vi "path steer7.vi"(11 "lane":bool) -> (2 "curve vel limit":dbl=3.2139390725243686, 3 "handle":dbl=-81.96459499192818)   [LabVIEW 2015]
uses:
  G_ALL.vi
  G_LCM.vi
  <vilib>/Analysis/polynomials.llb/Scalar Polynomial Evaluation (DBL).vi
  <vilib>/Analysis/polynomials.llb/nth Derivative of Polynomial (DBL).vi
  <vilib>/Analysis/polynomials.llb/1D Polynomial Evaluation (DBL).vi
  <vilib>/Analysis/NI_AALPro.lvlib
  G_SEN.vi
  <vilib>/gmath/NI_Gmath.lvlib
panel:
  out "Waveform Chart 2":dynamicdata(graph)
  in  "lpf gain 2":dbl=0.88 format="%#_13g"
  in  "parking stop":bool=TRUE
  out "cy":dbl
  out "cx":dbl
  out "slope ab":dbl
  out "slope bc":dbl
  out "current":i32
  in  "speed gain":dbl=0.3 format="%#_13g"
  in  "lpf gain":dbl=0.1 format="%#_13g"
  out "Waveform Chart":dbl(graph)=3.2139390725243686
  in  "index (row)":i32
  out "dist speed":dbl[](array[numeric])=[-2.893089960514653, -2.3904015790595508, -1.881068928132613, -1.37618634654772, -0.8742713561658589, -0.3723658755970851, 0.1388818221238658, 0.6401970171432404, 1.1461801054227339, 1.6534687725008643, 2.1616153665314632, 2.66800643713298, 3.175087235872203, 3.683904013545636, 4.1920491404702815, 4.703688631377526, 5.208864123676872, 5.719321128099619, 6.224971964952173, 6.729181230795628, 7.2363172303323795, 7.739934572021128, 8.247038660118557, 8.752204204665103, 9.255845634255843, 9.765210087355028, 10.274718584659908, 10.78117636416095, 11.281375299651366, 11.781461553901512, 12.293088227883759, 12.79457373850707, 13.302719176130964, 13.812473318001016, 14.318113179991025, 14.83081141605283, 15.340843713390877, 15.852065999952396, 16.364391250745, 16.8738363825444, 17.383376701480152, 17.890443538120152, 18.401927893044, 18.911251065570802, 19.420871980672878, 19.927741491376995, 20.442181893066248, 20.954251161353227, 21.455793255420453, 21.973813140636935, 22.47769405993468, 22.987685957840586, 23.50066957065988, 24.01168868408926, 24.517992353494144]
  out "Polynomial Coefficients 2":dbl[](array[numeric])
  out "R0":dbl=26.83387719970357
  out "handle 2":dbl=81.96459499192818
  out "dist":dbl[](array[numeric])=[-3.4007239355103813, -2.893089960514653, -2.3904015790595508, -1.881068928132613, -1.37618634654772, -0.8742713561658589, -0.3723658755970851, 0.1388818221238658, 0.6401970171432404, 1.1461801054227339, 1.6534687725008643, 2.1616153665314632, 2.66800643713298, 3.175087235872203, 3.683904013545636, 4.1920491404702815, 4.703688631377526, 5.208864123676872, 5.719321128099619, 6.224971964952173]
  in  "ap[g]":dbl=0.01 format="%#_13g"
  in  "mu":dbl=0.35 format="%#_13g"
  in  "an[g]":dbl=-0.03 format="%#_13g"
  out "Waveform Graph 2":dynamicdata(graph)=[{"t0"=timestamp(3559051319.3986335 s since 1904-01-01), "dt"=1.0, "Y"=[12.201099406852837, 18.19581647475159, 7.659888709456787, 6.442363646204152, 5.714419173702362, 7.179343934552439, 4.440534485019003, 4.39078441294489, 3.356713814067408, 2.401942511989647, 2.947435527157797, 2.405147000486268, 2.4253719977268635, 2.206819680096971, 2.0623492643882435, 1.9270030620983392, 1.8994447737647506, 1.8, 1.8, 1.8, 1.8, 1.8, 1.8, 2.1782596057309664, 2.252935408002384, 2.211867158231172, 2.2822368344295345, 2.820696071361234, 3.770354448612146, 2.5415686609617323, 9.592181945625502, 6.158409445479877, 5.390039216536413, 5.524972901149052, 13.273555614419179, 5.975286485301752, 11.57649163445339, 9.01145671123187, 9.660936533884865, 7.724510571264461, 5.533992586139264, 6.25966127157872, 14.880677288421989, 7.369567618162387, 13.568928447863307, 21.814825265892647, 18.32662456942843, 11.069099853071005, 65.39630065395748, 8.723651409692232, 11.138954896953177, 34.68633250782535, 14.254469597416035, 11.910088090354131, 13.122894121811795]}, {"t0"=timestamp(3559051319.3986335 s since 1904-01-01), "dt"=1.0, "Y"=[4.162943567044335, 4.006480657019834, 3.8414555364164134, 3.6705571026990116, 3.4923837272772165, 3.304621450941619, 3.101700634836984, 2.8889144351091893, 2.6569224873325505, 2.401942511989647, 2.659390719977461, 2.405147000486268, 2.4253719977268635, 2.206819680096971, 2.0623492643882435, 1.9270030620983392, 1.8994447737647506, 1.8, 1.8, 1.8, 1.8, 1.8, 1.8, 2.1782596057309664, 2.252935408002384, 2.211867158231172, 2.2822368344295345, 2.820696071361234, 2.780497542086646, 2.5415686609617323, 5.623145371472975, 5.508594247501762, 5.390039216536413, 5.524972901149052, 6.083396505782966, 5.975286485301752, 5.984875001532974, 5.8752716781758645, 5.763341152167903, 5.649841467554542, 5.533992586139264, 6.25966127157872, 7.456916882616871, 7.369567618162387, 9.088101570636532, 9.016914477587346, 8.944084767926125, 8.8709969665068, 8.798823217737656, 8.723651409692232, 11.138954896953177, 12.018901085380875, 11.964513913766247, 11.910088090354131, 13.122894121811795]}, {"t0"=timestamp(0 s since 1904-01-01), "dt"=1.0, "Y"=[4.162943567044335, 4.006480657019834, 3.8414555364164134, 3.6705571026990116, 3.4923837272772165, 3.304621450941619, 3.101700634836984, 2.8889144351091893, 2.6569224873325505, 2.401942511989647, 2.659390719977461, 2.405147000486268, 2.4253719977268635, 2.206819680096971, 2.0623492643882435, 1.9270030620983392, 1.8994447737647506, 1.8, 1.8, 1.8, 1.8, 1.8, 1.8, 2.1782596057309664, 2.252935408002384, 2.211867158231172, 2.2822368344295345, 2.820696071361234, 2.780497542086646, 2.5415686609617323, 5.623145371472975, 5.508594247501762, 5.390039216536413, 5.524972901149052, 6.083396505782966, 5.975286485301752, 5.984875001532974, 5.8752716781758645, 5.763341152167903, 5.649841467554542, 5.533992586139264, 6.25966127157872, 7.456916882616871, 7.369567618162387, 9.088101570636532, 9.016914477587346, 8.944084767926125, 8.8709969665068, 8.798823217737656, 8.723651409692232, 11.138954896953177, 12.018901085380875, 11.964513913766247, 11.910088090354131, 13.122894121811795]}]
  out "map_track for speed":dbl[][](array[numeric])=[[0.11349876041351359, -3.3998372416388567], [0.10142427488084116, -2.8923468876723155], [0.08838339602237211, -2.3898276897021793], [0.07566482613937353, -1.8806538615448463], [0.06028455243766717, -1.376005599516048], [0.0488631758884196, -0.8742205760969111], [0.04234520267579428, -0.3723574199973909], [0.038899869961946, 0.1388786684269922], [0.04370378366690808, 0.6401708458748642], [0.056953881218304414, 1.1459804153174877], [0.08472623749133856, 1.6525082901407298], [0.14087522942915354, 2.1575431916369188], [0.21546998499325254, 2.6584099791436198], [0.3179687305625989, 3.155023454199139], [0.44800644132001843, 3.6469428653052116], [0.6101750776411523, 4.128516123918072], [0.8099098158192999, 4.599558588055575], [1.0468148112307838, 5.045740502938923], [1.3255371094151536, 5.4733854887145865], [1.6426512363159849, 5.867240029541034], [1.9985777122494781, 6.224372116438809], [2.393384520275489, 6.5426715138030715], [2.816110574573037, 6.816410641199336], [3.267091466034361, 7.048295939788691], [3.738316452139705, 7.23033780274067], [4.219304825636487, 7.3796859669782116], [4.714356791323436, 7.499584663178458], [5.216398310074203, 7.586493939301898], [5.719828055076203, 7.641792892857529], [6.218830226700244, 7.6763733465884485], [6.718368390858731, 7.699780273749206], [7.229992817877207, 7.698263959746944], [7.731478256454141, 7.698532772738272], [8.239607735597689, 7.694505589692504], [8.749269272570775, 7.684789475041773], [9.254687125600576, 7.669807356632795], [9.767131481073555, 7.653674662971492], [10.277036204891097, 7.642267780992534], [10.788156814263154, 7.632072245090674], [11.300416991351074, 7.623906856578211], [11.809822584072345, 7.617559855837815], [12.319350308624628, 7.613977324090475], [12.826414003897163, 7.615762192897625], [13.337862856989585, 7.621788468887832], [13.847141338275545, 7.628535510597585], [14.35666821837679, 7.638325074620945], [14.8634605074283, 7.647172483245015], [15.377816289134199, 7.6565029020949416], [15.889810107971169, 7.665292953101379], [16.391253932531534, 7.675220839664499], [16.909171541171744, 7.685514145261032], [17.412991119838455, 7.6933762686663645], [17.92293988059403, 7.700009317250687], [18.43587828140128, 7.706819897140418], [18.946840832903064, 7.714422873724447], [19.45310431820556, 7.720801674725955], [19.97546574871732, 7.728375286190201]]
  out "Polynomial Coefficients":dbl[](array[numeric])=[0.03615792236483369, -0.0013391473415595393, 0.015775244563062195, 0.003058081181776752, 0.00017869743224815146, 3.406886139257993e-05]
  out "XY Graph":cluster{"Y":dbl[], "Y":dbl[]}[](graph)=[{"Y"=[0.11349876041351359, 0.10142427488084116, 0.08838339602237211, 0.07566482613937353, 0.06028455243766717, 0.0488631758884196, 0.04234520267579428, 0.038899869961946, 0.04370378366690808, 0.056953881218304414, 0.08472623749133856, 0.14087522942915354, 0.21546998499325254, 0.3179687305625989, 0.44800644132001843, 0.6101750776411523, 0.8099098158192999, 1.0468148112307838, 1.3255371094151536, 1.6426512363159849, 1.9985777122494781, 2.393384520275489, 2.816110574573037, 3.267091466034361, 3.738316452139705, 4.219304825636487, 4.714356791323436, 5.216398310074203, 5.719828055076203, 6.218830226700244, 6.718368390858731, 7.229992817877207, 7.731478256454141, 8.239607735597689, 8.749269272570775, 9.254687125600576, 9.767131481073555, 10.277036204891097, 10.788156814263154, 11.300416991351074, 11.809822584072345, 12.319350308624628, 12.826414003897163, 13.337862856989585, 13.847141338275545, 14.35666821837679, 14.8634605074283, 15.377816289134199, 15.889810107971169, 16.391253932531534, 16.909171541171744, 17.412991119838455, 17.92293988059403, 18.43587828140128, 18.946840832903064, 19.45310431820556, 19.97546574871732], "Y"=[-3.3998372416388567, -2.8923468876723155, -2.3898276897021793, -1.8806538615448463, -1.376005599516048, -0.8742205760969111, -0.3723574199973909, 0.1388786684269922, 0.6401708458748642, 1.1459804153174877, 1.6525082901407298, 2.1575431916369188, 2.6584099791436198, 3.155023454199139, 3.6469428653052116, 4.128516123918072, 4.599558588055575, 5.045740502938923, 5.4733854887145865, 5.867240029541034, 6.224372116438809, 6.5426715138030715, 6.816410641199336, 7.048295939788691, 7.23033780274067, 7.3796859669782116, 7.499584663178458, 7.586493939301898, 7.641792892857529, 7.6763733465884485, 7.699780273749206, 7.698263959746944, 7.698532772738272, 7.694505589692504, 7.684789475041773, 7.669807356632795, 7.653674662971492, 7.642267780992534, 7.632072245090674, 7.623906856578211, 7.617559855837815, 7.613977324090475, 7.615762192897625, 7.621788468887832, 7.628535510597585, 7.638325074620945, 7.647172483245015, 7.6565029020949416, 7.665292953101379, 7.675220839664499, 7.685514145261032, 7.6933762686663645, 7.700009317250687, 7.706819897140418, 7.714422873724447, 7.720801674725955, 7.728375286190201]}, {"Y"=[0.11127739316480087, 0.10361692506575307, 0.0908884914373908, 0.07556394971539812, 0.06037459789185977, 0.04742882065356524, 0.03868911291226688, 0.03628446458426678, 0.04260160497064784, 0.06031835031844553, 0.09257618876938067, 0.14288063799816245, 0.21498550882016326, 0.3133602690293894, 0.44300969189444267, 0.607484992736191, 0.8114301214735165, 1.0511320562375182, 1.3305918725474135, 1.6376613473029409, 1.9629799067769196, 2.2950444233922735, 2.6156651813619924, 2.9148313405818387, 3.1686664277537977, 3.3900852782615782, 3.576818603835668, 3.7173442133091044, 3.809077950572423, 3.867374654316165, 3.907246206986835, 3.9046531883929876, 3.905112777752115, 3.898232126569368, 3.8816723523358934, 3.856249915036759, 3.829027163652526, 3.809873646729178, 3.79282033229891, 3.779207635636962, 3.768653959202114, 3.762707611314233, 3.7656692101174953, 3.775682543110717, 3.786919264560898, 3.8032715749983694, 3.8180996271049827, 3.8337882452990133, 3.848616328842317, 3.865420072795456, 3.88290546839812, 3.8963043998905627, 3.9076380118640244, 3.9193029379730002, 3.932358601774901, 3.943339494877334, 3.9564096926462176], "Y"=[-3.3998372416388567, -2.8923468876723155, -2.3898276897021793, -1.8806538615448463, -1.376005599516048, -0.8742205760969111, -0.3723574199973909, 0.1388786684269922, 0.6401708458748642, 1.1459804153174877, 1.6525082901407298, 2.1575431916369188, 2.6584099791436198, 3.155023454199139, 3.6469428653052116, 4.128516123918072, 4.599558588055575, 5.045740502938923, 5.4733854887145865, 5.867240029541034, 6.224372116438809, 6.5426715138030715, 6.816410641199336, 7.048295939788691, 7.23033780274067, 7.3796859669782116, 7.499584663178458, 7.586493939301898, 7.641792892857529, 7.6763733465884485, 7.699780273749206, 7.698263959746944, 7.698532772738272, 7.694505589692504, 7.684789475041773, 7.669807356632795, 7.653674662971492, 7.642267780992534, 7.632072245090674, 7.623906856578211, 7.617559855837815, 7.613977324090475, 7.615762192897625, 7.621788468887832, 7.628535510597585, 7.638325074620945, 7.647172483245015, 7.6565029020949416, 7.665292953101379, 7.675220839664499, 7.685514145261032, 7.6933762686663645, 7.700009317250687, 7.706819897140418, 7.714422873724447, 7.720801674725955, 7.728375286190201]}]
  out "ref":dbl[](array[numeric])=[91.349795796563, 0.0013391465410557935, 0.021526577035807966]
  in  "gain":dbl[](array[numeric])=[0.7, -1400.0, 750.0]
  out "path end":bool
  out "map_track for steering":dbl[][](array[numeric])=[[0.11349876041351359, -3.3998372416388567], [0.10142427488084116, -2.8923468876723155], [0.08838339602237211, -2.3898276897021793], [0.07566482613937353, -1.8806538615448463], [0.06028455243766717, -1.376005599516048], [0.0488631758884196, -0.8742205760969111], [0.04234520267579428, -0.3723574199973909], [0.038899869961946, 0.1388786684269922], [0.04370378366690808, 0.6401708458748642], [0.056953881218304414, 1.1459804153174877], [0.08472623749133856, 1.6525082901407298], [0.14087522942915354, 2.1575431916369188], [0.21546998499325254, 2.6584099791436198], [0.3179687305625989, 3.155023454199139], [0.44800644132001843, 3.6469428653052116], [0.6101750776411523, 4.128516123918072], [0.8099098158192999, 4.599558588055575], [1.0468148112307838, 5.045740502938923], [1.3255371094151536, 5.4733854887145865], [1.6426512363159849, 5.867240029541034]]
  in  "control point":dbl=0.3 format="%#_13g"
  out "R_new":dbl=26.837045395498738
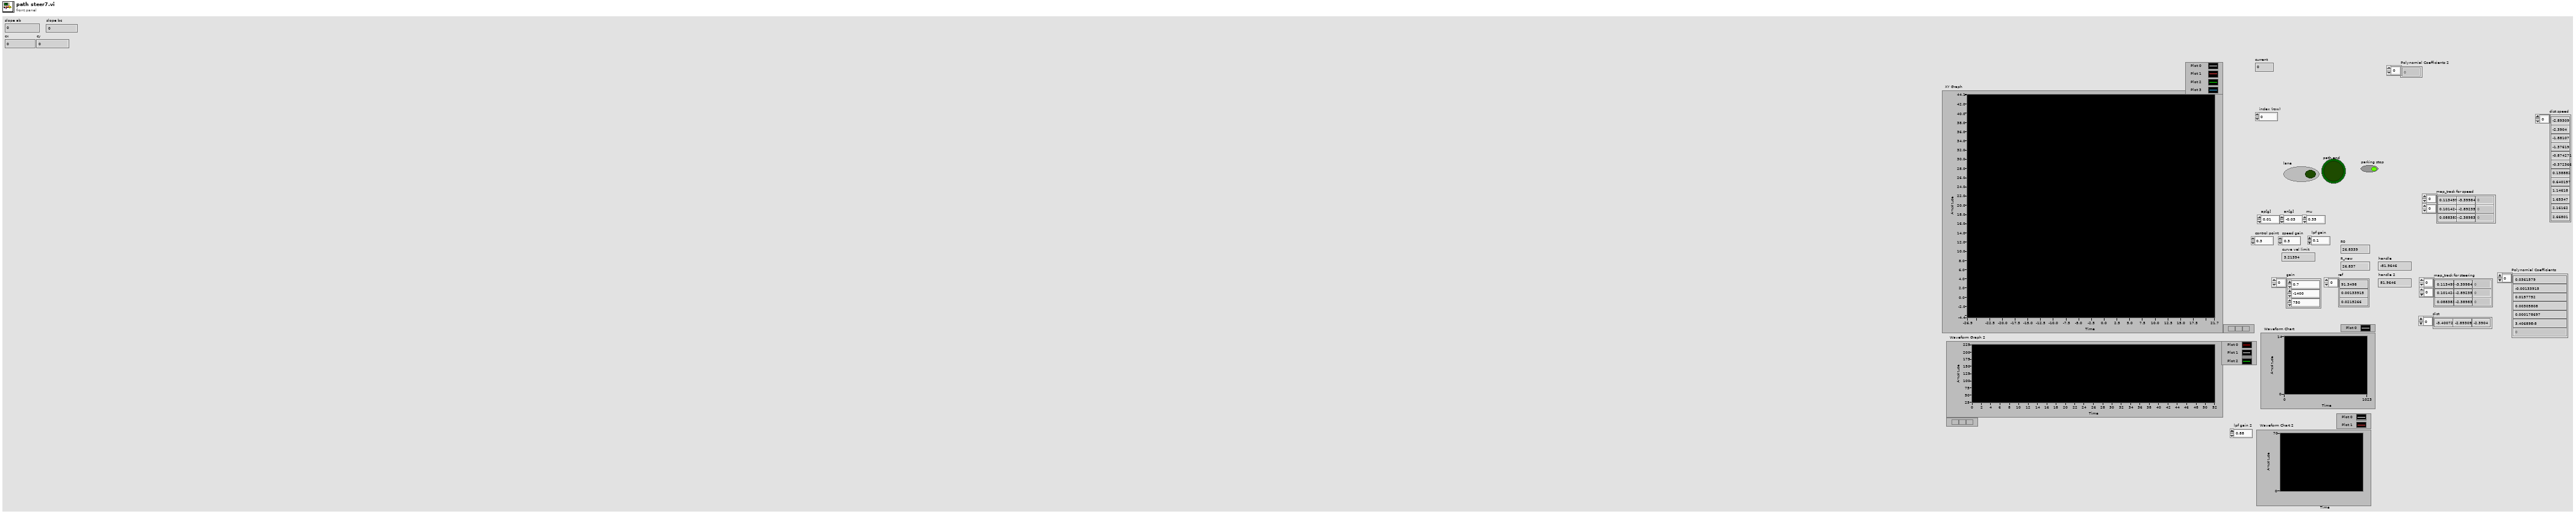
[diagram p1: front panel]
types:
  T1 = cluster{"Steer_input":dbl, "Steer_output":dbl, "VS_des":dbl, "VS_can":dbl, "heading":dbl, "auto":bool, "run":bool, "x":dbl, "y":dbl, "slam_y":dbl, "slam_x":dbl, "slam_heading":dbl}
  T2 = cluster{"C_Wheel base":dbl, "ratio_steer":dbl, "Overall width":dbl, "af":dbl, "turn radius":dbl, "eval":dbl, "ap":dbl, "an":dbl, "Vmax":dbl, "mu":dbl, "Vlast":dbl}
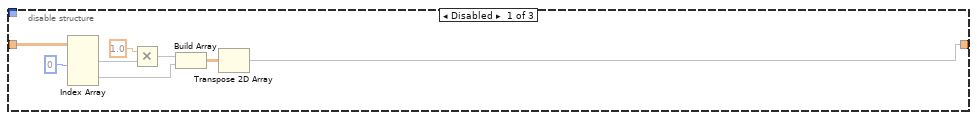
[diagram p2: hidden frame]
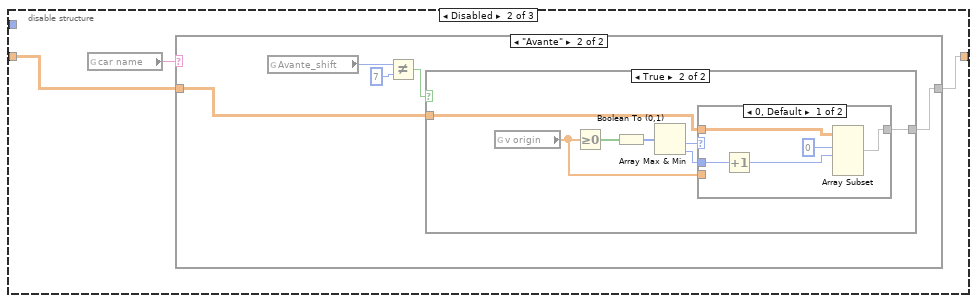
[diagram p3: hidden frame]
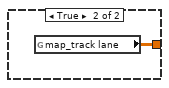
[diagram p7: hidden frame]
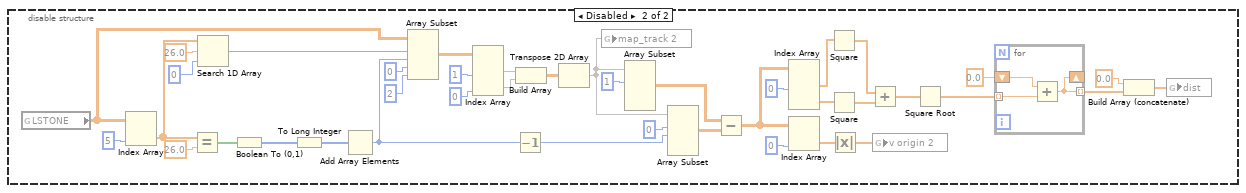
[diagram p8: hidden frame]
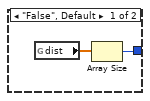
[diagram p11: hidden frame]
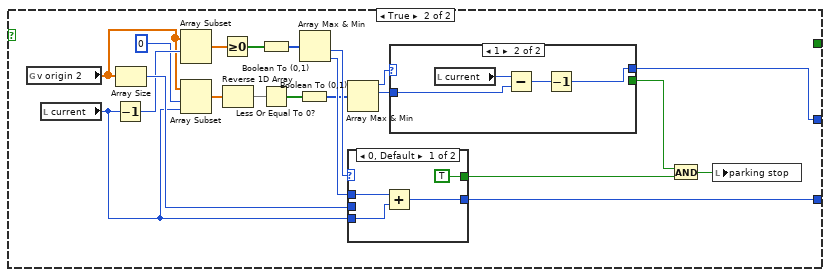
[diagram p13: hidden frame]
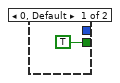
[diagram p14: hidden frame]
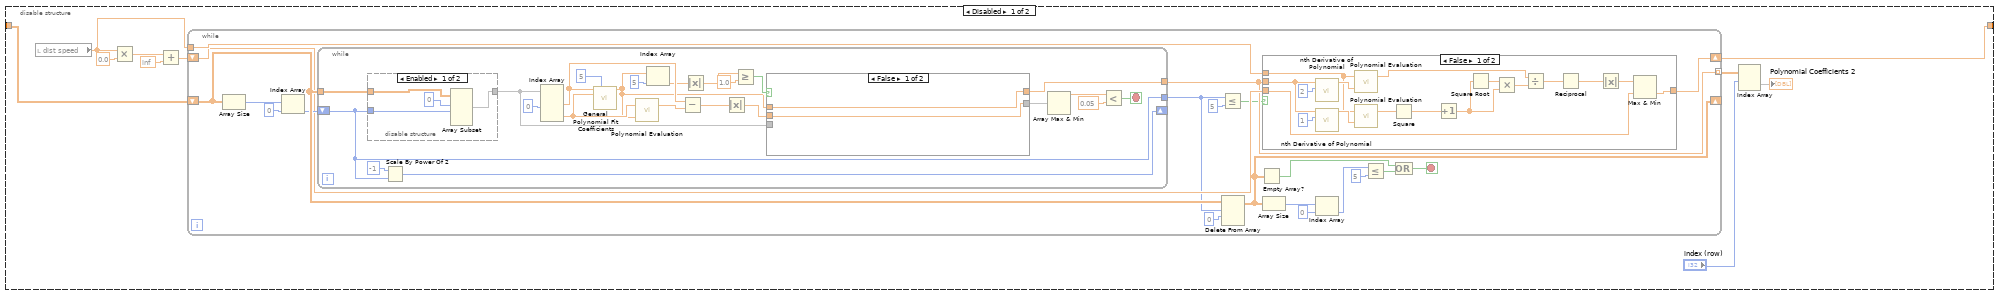
[diagram p16: hidden frame]
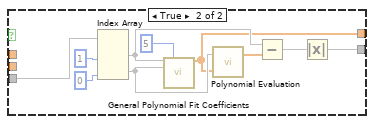
[diagram p18: hidden frame]
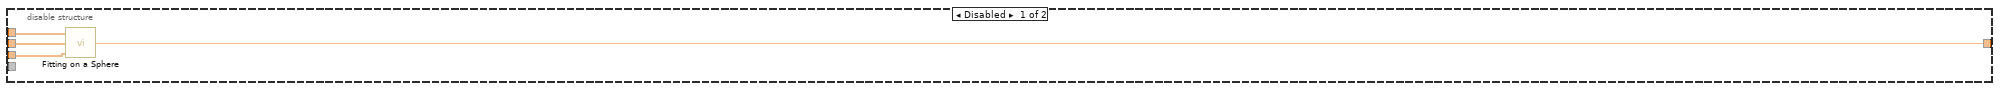
[diagram p20: hidden frame]
diagram:
  n1 = flat-sequence {
    tunnel: [w265] -> w2
    tunnel: w2 -> [w518]
    tunnel: [w633] -> w6
    tunnel: w6 -> [w644]
    tunnel: [w644] -> w5
    tunnel: [w638] -> w4
    tunnel: [w634] -> w3
    tunnel: [w635] -> w1
    tunnel: w5 -> [w696]
    tunnel: w4 -> [w694]
    tunnel: w3 -> [w675]
    tunnel: w1 -> [w671]
    frame #0 {
      n2 = disable-structure shown="Enabled" {
        frame Enabled {
          n3 = case shown="False" "lane" {
            tunnel: [w95 w138] -> w33
            tunnel: [w97 _] -> w66
            frame False {
              n4 = global read "G_ALL.vi" "current idx"() -> (w98:i32)
              n5 = Subtract(x=w98, y=2) -> (x-y=w105:i32)
              n6 = global read "G_ALL.vi" "map_track"() -> (w96:dbl[][])
              n7 = Max & Min(x=w105, y=0) -> (max(x,y)=w93:i32)  [unwired: 1 out]
              n8 = disable-structure shown="Enabled" {
                disable-tunnel: w96 -> [w114 w116 w137]
                disable-tunnel: [w107 w115 w137] -> w95
                disable-tunnel: w93 -> [_ _ _]
                frame Disabled {
                  n9 = Index Array(array=w114, index (col) #1=0 ("disabled index (col)")) -> (element #1=w112:dbl[], element #2=w109:dbl[])  [unwired: 3 in]
                  n10 = Multiply(x=1.0, y=w112) -> (x*y=w110:dbl[])
                  n11 = Build Array(w110, w109) -> (w108:dbl[][])
                  n12 = Transpose 2D Array(2D array=w108) -> (transposed array=w107:dbl[][])
                }
                frame Disabled {
                  n13 = global read "G_LCM.vi" "car name"() -> (w117:string)
                  n14 = case shown="\"Avante\"" w117 {
                    tunnel: [w118 w120] -> w115
                    tunnel: w116 -> [w118 w119]
                    frame Default {
                    }
                    frame "Avante" {
                      n15 = global read "G_ALL.vi" "Avante_shift"() -> (w122:u8)
                      n16 = Not Equal?(x=w122, y=u8 7) -> (x != y?=w121:bool)
                      n17 = case shown="True" w121 {
                        tunnel: [_ w126] -> w120
                        tunnel: w119 -> [_ w125]
                        frame False {
                        }
                        frame True {
                          n18 = global read "G_ALL.vi" "v origin"() -> (w127:dbl[])
                          n19 = Greater Or Equal To 0?(x=w127) -> (x >= 0?=w130:bool[])
                          n20 = Boolean To (0,1)(Boolean=w130) -> (0, 1=w129:i16[])
                          n21 = Array Max & Min(array=w129) -> (min value=w128:i16, min index (indices)=w124:i32)  [unwired: 2 out]
                          n22 = case shown="0, Default" w128 {
                            tunnel: w127 -> [_ _]
                            tunnel: [w132 w136] -> w126
                            tunnel: w125 -> [w134 w136]
                            tunnel: w124 -> [w135 _]
                            frame 0, Default {
                              n23 = Increment(x=w135) -> (x+1=w133:i32)
                              n24 = Array Subset(array=w134, index (row)=0 ("index"), length (row)=w133) -> (w132:dbl[][])  [unwired: 2 in]
                            }
                            frame 1 {
                            }
                          }
                        }
                      }
                    }
                  }
                }
                frame Enabled {
                }
              }
              n25 = Array Subset(array=w95, index (row)=w93, length (row)=5 ("length")) -> (w102:dbl[][])  [unwired: 2 in]
              n26 = Index Array(array=w102, index (col)=1 ("disabled index (col)")) -> (element=w100:dbl[])  [unwired: 1 in]
              n27 = Threshold 1D Array(2:0.0 ("threshold y"), 3:w100) -> (0:w94:dbl)  [unwired: 1 in]
              n28 = Add(x=w93, y=w94) -> (x+y=w97:dbl)
            }
            frame True {
              n29 = global read "G_ALL.vi" "map_track lane"() -> (w138:dbl[][])
            }
          }
          n30 = Round Toward -Infinity(1:w66) -> (0:w62:dbl)
          n31 = Index Array(array=w33, index (col) #1=0 ("disabled index (col)")) -> (element #1=w25:dbl[], element #2=w26:dbl[])  [unwired: 3 in]
          n32 = Equal?(x=w62, y=w66) -> (x = y?=w63:bool)
          n33 = To Long Integer(number=w62) -> (32bit integer=w64:i32)
          n34 = Interpolate 1D Array(1:w66, 2:w25) -> (0:w27:dbl)
          n35 = Interpolate 1D Array(1:w66, 2:w26) -> (0:w28:dbl)
          n36 = Increment(x=w64) -> (x+1=w65:i32)
          n37 = Round Toward +Infinity(x=w66) -> (ceil(x): smallest int >= x=w61:dbl)
          n38 = Select(t=w64, s=w63, f=w65) -> (s? t:f=w21:i32)
          n39 = global read "G_ALL.vi" "CARDATA"() -> (w31:T1)
          n40 = Array Subset(array=w33, index (row)=0 ("index"), length (row)=w21) -> (w35:dbl[][])  [unwired: 2 in]
          n41 = Unbundle By Name(w31) -> ("VS_can"=w67:dbl)
          n42 = Index Array(array=w35, index (col) #1=0 ("disabled index (col)")) -> (element #1=w37:dbl[], element #2=w38:dbl[])  [unwired: 3 in]
          n43 = Reverse 1D Array(array=w37) -> (reversed array=w39:dbl[])
          n44 = Reverse 1D Array(array=w38) -> (reversed array=w40:dbl[])
          n45 = Multiply(x=2.0, y=w67) -> (x*y=w68:dbl)
          n46 = Build Array(w39, w40) -> (w59:dbl[][])
          n47 = To Long Integer(number=w61) -> (32bit integer=w13:i32)
          n48 = Max & Min(x=w68, y=25.0) -> (max(x,y)=w32:dbl)  [unwired: 1 out]
          n49 = Array Subset(array=w33, index (row)=w13) -> (w57:dbl[][])  [unwired: 3 in]
          n50 = Transpose 2D Array(2D array=w59) -> (transposed array=w60:dbl[][])
          n51 = Build Array(w27, w28) -> (w42:dbl[])
          n52 = for {
            tunnel: w60 -> [w75] mode=indexing
            shift-right: [w75] -> _
            shift-left: w42 -> [w82]
            shift-right: [w74] -> _
            shift-left: 0.0 -> [w77]
            tunnel: 15.0 ("y") -> [w76]
            tunnel: [w74] -> w46 mode=indexing
            stop <- w73 stop-if-true
            n53 = Subtract(x=w75, y=w82) -> (x-y=w81:dbl[])
            n54 = Square(x=w81) -> (x^2=w80:dbl[])
            n55 = Add Array Elements(numeric array=w80) -> (sum=w79:dbl)
            n56 = Square Root(x=w79) -> (sqrt(x)=w78:dbl)
            n57 = Add(x=w77, y=w78) -> (x+y=w74:dbl)
            n58 = Greater Or Equal?(x=w74, y=w76) -> (x >= y?=w73:bool)
          }
          n59 = for {
            tunnel: w57 -> [w85] mode=indexing
            shift-right: [w85] -> _
            shift-left: w42 -> [w92]
            shift-right: [w84] -> _
            shift-left: 0.0 -> [w87]
            tunnel: w32 -> [w86]
            tunnel: [w84] -> w58 mode=indexing
            tunnel: [w83] -> w71
            stop <- w83 stop-if-true
            n60 = Subtract(x=w85, y=w92) -> (x-y=w91:dbl[])
            n61 = Square(x=w91) -> (x^2=w90:dbl[])
            n62 = Add Array Elements(numeric array=w90) -> (sum=w89:dbl)
            n63 = Square Root(x=w89) -> (sqrt(x)=w88:dbl)
            n64 = Add(x=w87, y=w88) -> (x+y=w84:dbl)
            n65 = Greater Or Equal?(x=w84, y=w86) -> (x >= y?=w83:bool)
          }
          n66 = global read "G_ALL.vi" "v origin"() -> (w14:dbl[])
          n67 = Array Subset(array=w14, index=0, length=w21) -> (w19:dbl[])
          n68 = Negate(x=w46) -> (-x=w44:dbl[])
          n69 = Not(x=w71) -> (.not. x?=→"path end":bool)
          n70 = Array Size(array=w46) -> (size(s)=w16:i32)
          n71 = Array Size(array=w58) -> (size(s)=w12:i32)
          n72 = Reverse 1D Array(array=w19) -> (reversed array=w18:dbl[])
          n73 = Array Subset(array=w14, index=w13, length=w12) -> (w11:dbl[])
          n74 = Reverse 1D Array(array=w44) -> (reversed array=w45:dbl[])
          n75 = Array Subset(array=w60, index (row)=0 ("index"), length (row)=w16) -> (w52:dbl[][])  [unwired: 2 in]
          n76 = Array Subset(array=w57, index (row)=0 ("index"), length (row)=w12) -> (w70:dbl[][])  [unwired: 2 in]
          n77 = Build Array (concatenate)(w45, w58) -> (w22:dbl[])
          n78 = Array Subset(array=w18, index=0, length=w16) -> (w15:dbl[])
          n79 = global write "G_ALL.vi" "dist"(w22) -> ()
          n80 = Reverse 1D Array(array=w15) -> (reversed array=w8:dbl[])
          n81 = Index Array(array=w52, index (col) #1=0 ("disabled index (col)")) -> (element #1=w53:dbl[], element #2=w54:dbl[])  [unwired: 3 in]
          n82 = Reverse 1D Array(array=w53) -> (reversed array=w50:dbl[])
          n83 = Reverse 1D Array(array=w54) -> (reversed array=w49:dbl[])
          n84 = Array Size(array=w8) -> (size(s)=→"current":i32)
          n85 = Build Array (concatenate)(w8, w11) -> (w10:dbl[])
          n86 = global write "G_ALL.vi" "v origin 2"(w10) -> ()
          n87 = Build Array(w50, w49) -> (w48:dbl[][])
          n88 = Transpose 2D Array(2D array=w48) -> (transposed array=w55:dbl[][])
          n89 = Build Array (concatenate)(w55, w70) -> (w23:dbl[][])
          n90 = global write "G_ALL.vi" "map_track 2"(w23) -> ()
        }
        frame Disabled {
          n91 = global read "G_SEN.vi" "LSTONE"() -> (w170:sgl[][])
          n92 = Index Array(array=w170, index (col)=5 ("disabled index (col)")) -> (element=w176:sgl[])  [unwired: 1 in]
          n93 = Equal?(x=w176, y=sgl 26.0 ("element")) -> (x = y?=w174:bool[])
          n94 = Search 1D Array(1D array=w176, element=sgl 26.0, start index (0)=0) -> (index of element=w169:i32)
          n95 = Boolean To (0,1)(Boolean=w174) -> (0, 1=w172:i16[])
          n96 = To Long Integer(number=w172) -> (32bit integer=w171:i32[])
          n97 = Add Array Elements(numeric array=w171) -> (sum=w165:i32)
          n98 = Array Subset(array=w170, index (row)=w169, length (row)=w165, index (col)=0 ("index"), length (col)=2 ("length")) -> (w142:sgl[][])
          n99 = Index Array(array=w142, index (col) #1=1 ("index (col)"), index (col) #2=0 ("index (col)")) -> (element #1=w144:sgl[], element #2=w139:sgl[])  [unwired: 2 in]
          n100 = Decrement(x=w165) -> (x-1=w164:i32)
          n101 = Build Array(w144, w139) -> (w143:sgl[][])
          n102 = Transpose 2D Array(2D array=w143) -> (transposed array=w141:sgl[][])
          n103 = global write "G_ALL.vi" "map_track 2"(w141) -> ()
          n104 = Array Subset(array=w141, index (row)=1 ("index")) -> (w161:sgl[][])  [unwired: 3 in]
          n105 = Array Subset(array=w141, index (row)=0 ("index"), length (row)=w164) -> (w162:sgl[][])  [unwired: 2 in]
          n106 = Subtract(x=w161, y=w162) -> (x-y=w149:sgl[][])
          n107 = Index Array(array=w149, index (col) #1=0 ("disabled index (col)")) -> (element #1=w159:sgl[], element #2=w158:sgl[])  [unwired: 3 in]
          n108 = Index Array(array=w149, index (col)=0 ("disabled index (col)")) -> (element=w147:sgl[])  [unwired: 1 in]
          n109 = Square(x=w159) -> (x^2=w156:sgl[])
          n110 = Square(x=w158) -> (x^2=w157:sgl[])
          n111 = Absolute Value(x=w147) -> (abs(x)=w146:sgl[])
          n112 = Add(x=w156, y=w157) -> (x+y=w155:sgl[])
          n113 = global write "G_ALL.vi" "v origin 2"(w146) -> ()
          n114 = Square Root(x=w155) -> (sqrt(x)=w154:sgl[])
          n115 = for {
            tunnel: w154 -> [w181] mode=indexing
            shift-right: [w179] -> _
            shift-left: sgl 0.0 -> [w180]
            tunnel: [w179] -> w152 mode=indexing
            n116 = Add(x=w180, y=w181) -> (x+y=w179:sgl)
          }
          n117 = Build Array (concatenate)(sgl 0.0, w152) -> (w150:sgl[])
          n118 = global write "G_ALL.vi" "dist"(w150) -> ()
        }
      }
    }
    frame #1 {
      n119 = disable-structure shown="Enabled" {
        disable-tunnel: [w208 _] -> w199
        frame Enabled {
          n120 = global read "G_LCM.vi" "car name"() -> (w208:string)
        }
        frame Disabled {
        }
      }
      n121 = case shown="\"Avante\"" w199 {
        tunnel: [w209 w214] -> w184
        tunnel: [_ w213] -> w195
        tunnel: [_ w211] -> w183
        frame "False", Default {
          n122 = global read "G_ALL.vi" "dist"() -> (w210:dbl[])
          n123 = Array Size(array=w210) -> (size(s)=w209:i32)
        }
        frame "Avante" {
          n124 = global read "G_ALL.vi" "Avante_shift"() -> (w215:u8)
          n125 = Not Equal?(x=w215, y=u8 7) -> (x != y?=w212:bool)
          n126 = case shown="False" w212 {
            tunnel: [w224 w252] -> w214
            tunnel: [w228 w237] -> w213
            tunnel: [w218 _] -> w211
            frame False {
              n127 = local write "parking stop"(FALSE ("parking stop")) -> ()
              n128 = global read "G_ALL.vi" "v origin 2"() -> (w230:dbl[])
              n129 = Less Or Equal To 0?(x=w230) -> (x <= 0?=w225:bool[])
              n130 = Array Size(array=w230) -> (size(s)=w229:i32)
              n131 = Boolean To (0,1)(Boolean=w225) -> (0, 1=w222:i16[])
              n132 = To Long Integer(number=w222) -> (32bit integer=w221:i32[])
              n133 = Array Max & Min(array=w222) -> (max value=w226:i16, max index (indices)=w227:i32)  [unwired: 2 out]
              n134 = Add Array Elements(numeric array=w221) -> (sum=w223:i32)
              n135 = global read "G_ALL.vi" "mission num"() -> (w220:i32)
              n136 = case shown="1" w226 {
                tunnel: w229 -> [w231 _]
                tunnel: [_ w233] -> w228
                tunnel: w227 -> [_ w233]
                tunnel: [w231 w232] -> w224
                tunnel: w223 -> [_ w232]
                frame 0, Default {
                }
                frame 1 {
                }
              }
              n137 = Equal?(x=w220, y=6) -> (x = y?=w218:bool)
            }
            frame True {
              n138 = global read "G_ALL.vi" "v origin 2"() -> (w246:dbl[])
              n139 = local read "current"() -> (w245:i32)
              n140 = Decrement(x=w245) -> (x-1=w248:i32)
              n141 = Array Size(array=w246) -> (size(s)=w253:i32)
              n142 = Array Subset(array=w246, index=w248) -> (w247:dbl[])  [unwired: 1 in]
              n143 = Array Subset(array=w246, index=0, length=w245) -> (w243:dbl[])
              n144 = Greater Or Equal To 0?(x=w247) -> (x >= 0?=w254:bool[])
              n145 = Reverse 1D Array(array=w243) -> (reversed array=w242:dbl[])
              n146 = Boolean To (0,1)(Boolean=w254) -> (0, 1=w251:i16[])
              n147 = Less Or Equal To 0?(x=w242) -> (x <= 0?=w241:bool[])
              n148 = Boolean To (0,1)(Boolean=w241) -> (0, 1=w240:i16[])
              n149 = Array Max & Min(array=w251) -> (min value=w250:i16, min index (indices)=w249:i32)  [unwired: 2 out]
              n150 = Array Max & Min(array=w240) -> (max value=w239:i16, max index (indices)=w238:i32)  [unwired: 2 out]
              n151 = case shown="0, Default" w250 {
                tunnel: w253 -> [_ w264]
                tunnel: [w261 w264] -> w252
                tunnel: w249 -> [w263 _]
                tunnel: w245 -> [w262 _]
                tunnel: [TRUE _] -> w234
                frame 0, Default {
                  n152 = Add(x=w263, y=w262) -> (x+y=w261:i32)
                }
                frame 1 {
                }
              }
              n153 = case shown="1" w239 {
                tunnel: w238 -> [_ w258]
                tunnel: [_ w256] -> w237
                tunnel: [TRUE _] -> w236
                frame 0, Default {
                }
                frame 1 {
                  n154 = local read "current"() -> (w259:i32)
                  n155 = Subtract(x=w259, y=w258) -> (x-y=w257:i32)
                  n156 = Decrement(x=w257) -> (x-1=w256:i32)
                }
              }
              n157 = And(x=w236, y=w234) -> (x .and. y?=w235:bool)
              n158 = local write "parking stop"(w235) -> ()
            }
          }
        }
      }
      n159 = global read "G_ALL.vi" "dist"() -> (w198:dbl[])
      n160 = Array Subset(array=w198, index=w195, length=w184) -> (w192:dbl[])
      n161 = Threshold 1D Array(2:-3.0 ("threshold y"), 3:w192) -> (0:w206:dbl)  [unwired: 1 in]
      n162 = Round Toward -Infinity(1:w206) -> (0:w188:dbl)
      n163 = global read "G_ALL.vi" "map_track 2"() -> (w197:dbl[][])
      n164 = Select(t=0.0, s=w183, f=w188) -> (s? t:f=w189:dbl)
      n165 = Array Subset(array=w197, index (row)=w195, length (row)=w184) -> (w196:dbl[][])  [unwired: 2 in]
      n166 = To Long Integer(number=w189) -> (32bit integer=w191:i32)
      n167 = Array Subset(array=w196, index (row)=w191) -> (w194:dbl[][])  [unwired: 3 in]
      n168 = Array Subset(array=w192, index=w191) -> (→"dist speed":dbl[])  [unwired: 1 in]
      n169 = disable-structure shown="Enabled" {
        disable-tunnel: w194 -> [w207 _]
        frame Enabled {
          "map_track for speed" <- w207
        }
        frame Disabled {
        }
      }
      n170 = Threshold 1D Array(1:w191, 2:6.0 ("threshold y"), 3:w192) -> (0:w203:dbl)
      n171 = Round Toward +Infinity(x=w203) -> (ceil(x): smallest int >= x=w202:dbl)
      n172 = To Long Integer(number=w202) -> (32bit integer=w204:i32)
      n173 = Subtract(x=w204, y=w191) -> (x-y=w205:i32)
      n174 = Increment(x=w205) -> (x+1=w186:i32)
      n175 = Select(t=w184, s=w183, f=w186) -> (s? t:f=w185:i32)
      n176 = Array Subset(array=w196, index (row)=w191, length (row)=w185) -> (→"map_track for steering":dbl[][])  [unwired: 2 in]
      n177 = Array Subset(array=w192, index=w191, length=w185) -> (→"dist":dbl[])
    }
    frame #2 {
      n178 = local read "map_track for speed"() -> (w266:dbl[][])
      n179 = disable-structure shown="Enabled" {
        disable-tunnel: w266 -> [w276 w358]
        disable-tunnel: [w270 w356] -> w265
        frame Disabled {
          n180 = local read "dist speed"() -> (w275:dbl[])
          n181 = Multiply(x=w275, y=0.0) -> (x*y=w273:dbl[])
          n182 = Add(x=w273, y=inf) -> (x+y=w271:dbl[])
          n183 = while {
            shift-right: [w287] -> _
            shift-left: w276 -> [w294]
            tunnel: w275 -> [w291]
            shift-right: [w288] -> w270
            shift-left: w271 -> [w290]
            tunnel: [w289] -> w269 mode=indexing
            stop <- w281 stop-if-true
            n184 = Array Size(array=w294) -> (size(s)=w296:i32[])
            n185 = Index Array(array=w296, index=0) -> (element=w292:i32)
            n186 = while {
              tunnel: w294 -> [w331]
              shift-right: [w329] -> _
              shift-left: w292 -> [w325]
              tunnel: [w325] -> w277
              tunnel: [w318] -> w289
              stop <- w327 stop-if-true
              n187 = disable-structure shown="Enabled" {
                disable-tunnel: w331 -> [w352 w354]
                disable-tunnel: [w351 w354] -> w324
                disable-tunnel: w325 -> [w350 _]
                frame Enabled {
                  n188 = Array Subset(array=w352, index (row)=0 ("index"), length (row)=w350) -> (w351:dbl[][])  [unwired: 2 in]
                }
                frame Disabled {
                }
              }
              n189 = Scale By Power Of 2(n=i16 -1, x=w325) -> (x*2^n=w329:i32)
              n190 = Index Array(array=w324, index (col) #1=0 ("disabled index (col)")) -> (element #1=w335:dbl[], element #2=w333:dbl[])  [unwired: 3 in]
              n191 = call <vilib>:"General Polynomial Fit Coefficients.vi"("Y"=w335, "polynomial order"=5, "X"=w333) -> ("Polynomial Coefficients"=w317:dbl[])  [unwired: 11 in, 1 out]
              n192 = call-poly <vilib>:"Polynomial Evaluation.vi"("P(x)"=w317, "A"=w333) -> ("P(A)"=w332:dbl[])  [unwired: 1 out]
              n193 = Index Array(array=w317, index=5) -> (element=w316:dbl)
              n194 = Subtract(x=w335, y=w332) -> (x-y=w334:dbl[])
              n195 = Absolute Value(x=w316) -> (abs(x)=w315:dbl)
              n196 = Absolute Value(x=w334) -> (abs(x)=w319:dbl[])
              n197 = Greater Or Equal?(x=w315, y=1.0) -> (x >= y?=w321:bool)
              n198 = case shown="False" w321 {
                tunnel: w324 -> [_ w343]
                tunnel: [w339 w341] -> w320
                tunnel: w319 -> [w339 _]
                tunnel: [w338 w340] -> w318
                tunnel: w317 -> [w338 _]
                frame False {
                }
                frame True {
                  n199 = Index Array(array=w343, index (col) #1=1 ("disabled index (col)"), index (col) #2=0 ("index (col)")) -> (element #1=w346:dbl[], element #2=w348:dbl[])  [unwired: 2 in]
                  n200 = call <vilib>:"General Polynomial Fit Coefficients.vi"("Y"=w346, "polynomial order"=5, "X"=w348) -> ("Polynomial Coefficients"=w340:dbl[])  [unwired: 11 in, 1 out]
                  n201 = call-poly <vilib>:"Polynomial Evaluation.vi"("P(x)"=w340, "A"=w348) -> ("P(A)"=w349:dbl[])  [unwired: 1 out]
                  n202 = Subtract(x=w346, y=w349) -> (x-y=w347:dbl[])
                  n203 = Absolute Value(x=w347) -> (abs(x)=w341:dbl[])
                }
              }
              n204 = Array Max & Min(array=w320) -> (max value=w328:dbl)  [unwired: 3 out]
              n205 = Less?(x=w328, y=0.05) -> (x < y?=w327:bool)
            }
            n206 = Less Or Equal?(x=w277, y=5) -> (x <= y?=w278:bool)
            n207 = Delete From Array(array=w294, length=w277, index (row)=0) -> (array with subset deleted=w287:dbl[][])  [unwired: 1 in, 1 out]
            n208 = Empty Array?(array=w287) -> (empty?=w283:bool)
            n209 = case shown="False" w278 {
              tunnel: w291 -> [w302 _]
              tunnel: w290 -> [w300 w314]
              tunnel: w289 -> [w298 _]
              tunnel: [w297 w314] -> w288
              frame False {
                n210 = call-poly <vilib>:"nth Derivative of Polynomial.vi"("order"=2, "P(x)"=w298) -> ("Nth Derivative of P(x)"=w305:dbl[])  [unwired: 8 in, 1 out]
                n211 = call-poly <vilib>:"nth Derivative of Polynomial.vi"("order"=1, "P(x)"=w298) -> ("Nth Derivative of P(x)"=w307:dbl[])  [unwired: 8 in, 1 out]
                n212 = call-poly <vilib>:"Polynomial Evaluation.vi"("P(x)"=w305, "A"=w302) -> ("P(A)"=w303:dbl[])  [unwired: 1 out]
                n213 = call-poly <vilib>:"Polynomial Evaluation.vi"("P(x)"=w307, "A"=w302) -> ("P(A)"=w311:dbl[])  [unwired: 1 out]
                n214 = Square(x=w311) -> (x^2=w308:dbl[])
                n215 = Increment(x=w308) -> (x+1=w310:dbl[])
                n216 = Square Root(x=w310) -> (sqrt(x)=w309:dbl[])
                n217 = Multiply(x=w309, y=w310) -> (x*y=w306:dbl[])
                n218 = Divide(x=w303, y=w306) -> (x/y=w313:dbl[])
                n219 = Reciprocal(x=w313) -> (1/x=w301:dbl[])
                n220 = Absolute Value(x=w301) -> (abs(x)=w299:dbl[])
                n221 = Max & Min(x=w299, y=w300) -> (min(x,y)=w297:dbl[])  [unwired: 1 out]
              }
              frame True {
              }
            }
            n222 = Array Size(array=w287) -> (size(s)=w286:i32[])
            n223 = Index Array(array=w286, index=0) -> (element=w280:i32)
            n224 = Less Or Equal?(x=w280, y=5) -> (x <= y?=w282:bool)
            n225 = Compound Arithmetic op=OR(w283, w282) -> (w281:bool)
          }
          n226 = Index Array(array=w269, index (row)="index (row)") -> (element=→"Polynomial Coefficients 2":dbl[])  [unwired: 1 in]
        }
        frame Enabled {
          n227 = Array Size(array=w358) -> (size(s)=w364:i32[])
          n228 = Index Array(array=w364, index=0) -> (element=w362:i32)
          n229 = local read "dist speed"() -> (w360:dbl[])
          n230 = Subtract(x=w362, y=2) -> (x-y=w355:i32)
          n231 = for {
            N: w355 -> [_]
            tunnel: w358 -> [w377]
            tunnel: [w370] -> w357 mode=indexing
            tunnel: w360 -> [w369]
            tunnel: [w366] -> w359 mode=indexing
            i -> [w368]
            n232 = Increment(x=w368) -> (x+1=w367:i32)
            n233 = Array Subset(array=w377, index (row)=w368, length (row)=3 ("length")) -> (w365:dbl[][])  [unwired: 2 in]
            n234 = Index Array(array=w369, index=w367) -> (element=w366:dbl)
            n235 = Index Array(array=w365, index (col) #1=0 ("disabled index (col)")) -> (element #1=w374:dbl[], element #2=w373:dbl[])  [unwired: 3 in]
            n236 = Multiply(x=w373, y=0.0) -> (x*y=w372:dbl[])
            n237 = disable-structure shown="Enabled" {
              disable-tunnel: w374 -> [w381 _]
              disable-tunnel: w373 -> [w380 _]
              disable-tunnel: w372 -> [w379 _]
              disable-tunnel: [w378 w382] -> w370
              disable-tunnel: w365 -> [_ w383]
              frame Disabled {
                n238 = call <vilib>:"Fitting on a Sphere.vi"("Z"=w379, "Y"=w380, "X"=w381) -> ("r"=w378:dbl)  [unwired: 2 out]
              }
              frame Enabled {
                n239 = flat-sequence {
                  tunnel: w383 -> [w392]
                  tunnel: [w392] -> w386
                  tunnel: w386 -> [w410]
                  tunnel: [w410] -> w385
                  tunnel: w385 -> [w442]
                  tunnel: [w442] -> w384
                  tunnel: w384 -> [w483]
                  tunnel: [w463] -> w382
                  tunnel: [w464] -> _
                  frame #0 {
                    n240 = Index Array(array=w392, index (col) #1=1 ("disabled index (col)"), index (col) #2=0 ("index (col)")) -> (element #1=w387:dbl[], element #2=w399:dbl[])  [unwired: 2 in]
                    n241 = Index Array(array=w387, index #1=0 ("index"), index #2=1 ("index"), index #3=2 ("index")) -> (element #1=w406:dbl, element #2=w405:dbl, element #3=w404:dbl)
                    n242 = Index Array(array=w399, index #1=0 ("index"), index #2=1 ("index"), index #3=2 ("index")) -> (element #1=w401:dbl, element #2=w402:dbl, element #3=w403:dbl)
                    n243 = Subtract(x=w406, y=w405) -> (x-y=w398:dbl)
                    n244 = Subtract(x=w405, y=w404) -> (x-y=w396:dbl)
                    n245 = Subtract(x=w401, y=w402) -> (x-y=w397:dbl)
                    n246 = Subtract(x=w402, y=w403) -> (x-y=w395:dbl)
                    n247 = Divide(x=w398, y=w397) -> (x/y=→"slope ab":dbl)
                    n248 = Divide(x=w396, y=w395) -> (x/y=→"slope bc":dbl)
                  }
                  frame #1 {
                    n249 = Index Array(array=w410, index (col) #1=0 ("disabled index (col)"), index (col) #2=1 ("index (col)")) -> (element #1=w440:dbl[], element #2=w427:dbl[])  [unwired: 2 in]
                    n250 = Index Array(array=w427, index #1=2 ("index"), index #2=0 ("index")) -> (element #1=w424:dbl, element #2=w423:dbl)
                    n251 = Index Array(array=w440, index #1=2 ("index"), index #2=1 ("index"), index #3=0 ("index")) -> (element #1=w435:dbl, element #2=w432:dbl, element #3=w431:dbl)
                    n252 = Subtract(x=w424, y=w423) -> (x-y=w414:dbl)
                    n253 = local read "slope ab"() -> (w434:dbl)
                    n254 = local read "slope bc"() -> (w413:dbl)
                    n255 = local read "slope ab"() -> (w412:dbl)
                    n256 = local read "slope bc"() -> (w421:dbl)
                    n257 = Add(x=w435, y=w432) -> (x+y=w433:dbl)
                    n258 = Add(x=w432, y=w431) -> (x+y=w430:dbl)
                    n259 = Multiply(x=w434, y=w433) -> (x*y=w429:dbl)
                    n260 = Multiply(x=w430, y=w413) -> (x*y=w428:dbl)
                    n261 = Subtract(x=w412, y=w421) -> (x-y=w420:dbl)
                    n262 = Compound Arithmetic op=MULTIPLY(w413, w414, w412) -> (w411:dbl)
                    n263 = Subtract(x=w429, y=w428) -> (x-y=w422:dbl)
                    n264 = Multiply(x=w420, y=2.0) -> (x*y=w417:dbl)
                    n265 = Add(x=w422, y=w411) -> (x+y=w418:dbl)
                    n266 = Divide(x=w418, y=w417) -> (x/y=→"cx":dbl)
                  }
                  frame #2 {
                    n267 = Index Array(array=w442, index (col) #1=0 ("index (row)")) -> (element #1=w461:dbl[], element #2=w446:dbl[])  [unwired: 3 in]
                    n268 = Index Array(array=w461, index #1=0 ("index")) -> (element #1=w459:dbl, element #2=w458:dbl)  [unwired: 1 in]
                    n269 = Index Array(array=w446, index #1=0 ("index")) -> (element #1=w448:dbl, element #2=w449:dbl)  [unwired: 1 in]
                    n270 = Add(x=w459, y=w458) -> (x+y=w457:dbl)
                    n271 = Add(x=w448, y=w449) -> (x+y=w450:dbl)
                    n272 = Multiply(x=w457, y=0.5) -> (x*y=w455:dbl)
                    n273 = local read "slope ab"() -> (w462:dbl)
                    n274 = local read "cx"() -> (w454:dbl)
                    n275 = Subtract(x=w455, y=w454) -> (x-y=w453:dbl)
                    n276 = Reciprocal(x=w462) -> (1/x=w452:dbl)
                    n277 = Multiply(x=w452, y=w453) -> (x*y=w445:dbl)
                    n278 = Multiply(x=w450, y=0.5) -> (x*y=w444:dbl)
                    n279 = Add(x=w445, y=w444) -> (x+y=→"cy":dbl)
                  }
                  frame #3 {
                    n280 = local read "cx"() -> (w477:dbl)
                    n281 = Index Array(array=w483, index (row)=0) -> (element=w478:dbl[])  [unwired: 1 in]
                    n282 = Sign(1:w477) -> (0:w476:dbl)
                    n283 = local read "cy"() -> (w481:dbl)
                    n284 = Build Array(w477, w481) -> (w474:dbl[])
                    n285 = Subtract(x=w474, y=w478) -> (x-y=w480:dbl[])
                    n286 = local read "cx"() -> (w472:dbl)
                    n287 = local read "cy"() -> (w471:dbl)
                    n288 = Square(x=w480) -> (x^2=w479:dbl[])
                    n289 = Square(x=w472) -> (x^2=w470:dbl)
                    n290 = Square(x=w471) -> (x^2=w469:dbl)
                    n291 = Add(x=w470, y=w469) -> (x+y=w468:dbl)
                    n292 = Add Array Elements(numeric array=w479) -> (sum=w467:dbl)
                    n293 = Subtract(x=w468, y=w467) -> (x-y=w466:dbl)
                    n294 = Square Root(x=w467) -> (sqrt(x)=w475:dbl)
                    n295 = Multiply(x=w474, y=-2.0) -> (x*y=w465:dbl[])
                    n296 = Multiply(x=w476, y=w475) -> (x*y=w463:dbl)
                    n297 = Build Array (concatenate)(w465, w466) -> (w464:dbl[])
                  }
                }
              }
            }
          }
          n298 = Absolute Value(x=w357) -> (abs(x)=w356:dbl[])
          n299 = local write "dist speed"(w359) -> ()
        }
      }
    }
    frame #3 {
      n300 = Compound Arithmetic op=MULTIPLY(w518, 9.81 ("value"), "mu") -> (w530:dbl[])
      n301 = Square Root(x=w530) -> (sqrt(x)=w516:dbl[])
      n302 = local read "path end"() -> (w490:bool)
      n303 = In Range and Coerce(upper limit=56.0 ("value"), x=w516, lower limit=0.5) -> (coerced(x)=w517:dbl[])  [unwired: 1 out]
      n304 = Or(x=w490, y="parking stop") -> (x .or. y?=w489:bool)
      n305 = Reverse 1D Array(array=w517) -> (reversed array=w537:dbl[])
      n306 = call "Convert to Dynamic Data6"("Array"=w517) -> ("Dynamic Data Type"=w521:dynamicdata)  [unwired: 3 in]
      n307 = case shown="True" w489 {
        tunnel: w537 -> [w603 w607]
        tunnel: [w603 w606] -> w538
        frame False {
        }
        frame True {
          n308 = Replace Array Subset(array=w607, new element=0.0 ("new element/subarray"), index=0) -> (w606:dbl[])
        }
      }
      n309 = local read "dist speed"() -> (w519:dbl[])
      n310 = Array Size(array=w538) -> (size(s)=w535:i32)
      n311 = Reverse 1D Array(array=w519) -> (reversed array=w532:dbl[])
      n312 = Decrement(x=w535) -> (x-1=w534:i32)
      n313 = Negate(x=w532) -> (-x=w533:dbl[])
      n314 = for {
        N: w534 -> [_]
        tunnel: w538 -> [w623] mode=indexing
        tunnel: w533 -> [w624]
        shift-right: [w614] -> w523
        shift-left: w538 -> [w617]
        tunnel: w533 -> [w611] mode=indexing
        tunnel: "an[g]" -> [w608]
        i -> [w625]
        n315 = Square(x=w623) -> (x^2=w622:dbl)
        n316 = Increment(x=w625) -> (x+1=w616:i32)
        n317 = Array Subset(array=w617, index=w616) -> (w618:dbl[])  [unwired: 1 in]
        n318 = Array Subset(array=w624, index=w616) -> (w612:dbl[])  [unwired: 1 in]
        n319 = Subtract(x=w612, y=w611) -> (x-y=w610:dbl[])
        n320 = Compound Arithmetic op=MULTIPLY(w610, 9.81 ("value"), 2.0 ("value"), w608) -> (w620:dbl[])
        n321 = Subtract(x=w622, y=w620) -> (x-y=w619:dbl[])
        n322 = Square Root(x=w619) -> (sqrt(x)=w613:dbl[])
        n323 = Max & Min(x=w618, y=w613) -> (min(x,y)=w615:dbl[])  [unwired: 1 out]
        n324 = Replace Array Subset(array=w617, new element=w615, index=w616) -> (w614:dbl[])
      }
      n325 = global read "G_ALL.vi" "mission num"() -> (w497:i32)
      n326 = case shown="6" w497 {
        tunnel: [1.0 w549] -> w496
        frame 0, Default {
        }
        frame 6 {
          n327 = global read "G_LCM.vi" "car name"() -> (w548:string)
          n328 = case shown="\"Avante\"" w548 {
            tunnel: [w550 w553] -> w547
            frame Default {
              n329 = global read "G_ALL.vi" "CARDATA"() -> (w552:T1)
              n330 = Unbundle By Name(w552) -> ("VS_can"=w551:dbl)
              n331 = Less Than 0?(x=w551) -> (x < 0?=w550:bool)
            }
            frame "Avante" {
              n332 = global read "G_ALL.vi" "Avante_shift"() -> (w554:u8)
              n333 = Equal?(x=w554, y=u8 7) -> (x = y?=w553:bool)
            }
          }
          n334 = case shown="True" w547 {
            tunnel: [w559 w570] -> w549
            tunnel: 0.1 -> [w556 w569]
            frame False {
              n335 = local read "map_track for steering"() -> (w562:dbl[][])
              n336 = Index Array(array=w562, index (col)=1 ("disabled index (col)")) -> (element=w564:dbl[])  [unwired: 1 in]
              n337 = Array Max & Min(array=w564) -> (max value=w558:dbl)  [unwired: 3 out]
              n338 = Less?(x=w558, y=w556) -> (x < y?=w557:bool)
              n339 = case shown="True" w557 {
                frame False {
                }
                frame True {
                  n340 = global write "G_ALL.vi" "Reverse"(TRUE ("Reverse")) -> ()
                }
              }
              n341 = Select(t=-1.0, s=w557, f=1.0) -> (s? t:f=w559:dbl)
            }
            frame True {
              n342 = Negate(x=w569) -> (-x=w567:dbl)
              n343 = local read "map_track for steering"() -> (w573:dbl[][])
              n344 = Index Array(array=w573, index (col)=1 ("disabled index (col)")) -> (element=w575:dbl[])  [unwired: 1 in]
              n345 = Array Max & Min(array=w575) -> (min value=w568:dbl)  [unwired: 3 out]
              n346 = Greater?(x=w568, y=w567) -> (0:w566:bool)
              n347 = case shown="True" w566 {
                frame False {
                }
                frame True {
                  n348 = global write "G_ALL.vi" "Reverse"(FALSE ("Reverse")) -> ()
                }
              }
              n349 = Select(t=1.0, s=w566, f=-1.0) -> (s? t:f=w570:dbl)
            }
          }
        }
      }
      n350 = Reverse 1D Array(array=w523) -> (reversed array=w510:dbl[])
      n351 = disable-structure shown="Enabled" {
        disable-tunnel: [w579 w602] -> w511
        disable-tunnel: w510 -> [w578 w602]
        frame Disabled {
          n352 = Array Size(array=w578) -> (size(s)=w582:i32)
          n353 = local read "dist speed"() -> (w577:dbl[])
          n354 = Decrement(x=w582) -> (x-1=w583:i32)
          n355 = Negate(x=w577) -> (-x=w580:dbl[])
          n356 = for {
            N: w583 -> [_]
            tunnel: w578 -> [w599] mode=indexing
            tunnel: w580 -> [w600]
            shift-right: [w590] -> w579
            shift-left: w578 -> [w593]
            tunnel: w580 -> [w587] mode=indexing
            tunnel: "ap[g]" -> [w584]
            i -> [w601]
            n357 = Square(x=w599) -> (x^2=w598:dbl)
            n358 = Increment(x=w601) -> (x+1=w592:i32)
            n359 = Array Subset(array=w593, index=w592) -> (w594:dbl[])  [unwired: 1 in]
            n360 = Array Subset(array=w600, index=w592) -> (w588:dbl[])  [unwired: 1 in]
            n361 = Subtract(x=w588, y=w587) -> (x-y=w586:dbl[])
            n362 = Compound Arithmetic op=MULTIPLY(w586, 9.81 ("value"), 2.0 ("value"), w584) -> (w596:dbl[])
            n363 = Subtract(x=w598, y=w596) -> (x-y=w595:dbl[])
            n364 = Square Root(x=w595) -> (sqrt(x)=w589:dbl[])
            n365 = Max & Min(x=w594, y=w589) -> (min(x,y)=w591:dbl[])  [unwired: 1 out]
            n366 = Replace Array Subset(array=w593, new element=w591, index=w592) -> (w590:dbl[])
          }
        }
        frame Enabled {
        }
      }
      n367 = call "Convert to Dynamic Data5"("Array"=w510) -> ("Dynamic Data Type"=w520:dynamicdata)  [unwired: 3 in]
      n368 = global read "G_LCM.vi" "car name"() -> (w486:string)
      n369 = case shown="Default" w486 {
        tunnel: [w539 w542] -> w488
        frame Default {
          n370 = global read "G_ALL.vi" "CARDATA"() -> (w541:T1)
          n371 = Unbundle By Name(w541) -> ("VS_can"=w540:dbl)
          n372 = Less Than 0?(x=w540) -> (x < 0?=w539:bool)
        }
        frame "Avante" {
          n373 = global read "G_ALL.vi" "Avante_shift"() -> (w544:u8)
          n374 = Equal?(x=w544, y=u8 7) -> (x = y?=w542:bool)
        }
      }
      n375 = local read "control point"() -> (w485:dbl)
      n376 = Negate(x=w485) -> (-x=w487:dbl)
      n377 = local read "dist speed"() -> (w512:dbl[])
      n378 = Select(t=w487, s=w488, f=w485) -> (s? t:f=w484:dbl)
      n379 = Threshold 1D Array(2:w484, 3:w512) -> (0:w528:dbl)  [unwired: 1 in]
      n380 = call "Convert to Dynamic Data7"("Array"=w511) -> ("Dynamic Data Type"=w524:dynamicdata)  [unwired: 3 in]
      n381 = Interpolate 1D Array(1:w528, 2:w511) -> (0:w499:dbl)
      n382 = Not A Number/Path/Refnum?(number/path/refnum=w499) -> (NaN/Path/Refnum?=w501:bool)
      n383 = Merge Signals(w521, w520, w524) -> (w526:dynamicdata)
      n384 = Select(t=0.0, s=w501, f=w499) -> (s? t:f=w498:dbl)
      n385 = Multiply(x=w526, y=3.6) -> (x*y=→"Waveform Graph 2":dynamicdata)
      n386 = Decrement(x="lpf gain") -> (x-1=w507:dbl)
      n387 = Multiply(x=w498, y=3.6) -> (x*y=w509:dbl)
      n388 = Multiply(x=w509, y="lpf gain") -> (x*y=w505:dbl)
      n389 = feedback #1(0.0) -> (w506:dbl)
      n390 = Multiply(x=w507, y=w506) -> (x*y=w504:dbl)
      n391 = Subtract(x=w505, y=w504) -> (x-y=w502:dbl)
      n392 = feedback-in #1(w502) -> ()
      n393 = Multiply(x=w502, y="speed gain") -> (x*y=w495:dbl)
      "Waveform Chart" <- w495
      n394 = Multiply(x=w495, y=w496) -> (x*y=w494:dbl)
      n395 = Max & Min(x=w494, y=-2.0) -> (max(x,y)=→"curve vel limit":dbl)  [unwired: 1 out]
    }
    frame #4 {
      n396 = local read "map_track for steering"() -> (w632:dbl[][])
      n397 = Index Array(array=w632, index (col) #1=0 ("disabled index (col)")) -> (element #1=w629:dbl[], element #2=w630:dbl[])  [unwired: 3 in]
      n398 = call <vilib>:"General Polynomial Fit Coefficients.vi"("Y"=w629, "polynomial order"=5, "X"=w630) -> ("Polynomial Coefficients"=w626:dbl[])  [unwired: 11 in, 1 out]
      "Polynomial Coefficients" <- w626
      n399 = call-poly <vilib>:"Polynomial Evaluation.vi"("P(x)"=w626, "a"=0.0) -> ("P(a)"=w633:dbl)  [unwired: 1 out]
    }
    frame #5 {
      n400 = global read "G_LCM.vi" "car name"() -> (w640:string)
      n401 = case shown="Default" w640 {
        tunnel: [w655 w658] -> w634
        frame Default {
          n402 = global read "G_ALL.vi" "CARDATA"() -> (w657:T1)
          n403 = Unbundle By Name(w657) -> ("VS_can"=w656:dbl)
          n404 = Less Than 0?(x=w656) -> (x < 0?=w655:bool)
        }
        frame "Avante" {
          n405 = global read "G_ALL.vi" "Avante_shift"() -> (w660:u8)
          n406 = Equal?(x=w660, y=u8 7) -> (x = y?=w658:bool)
        }
      }
      n407 = Negate(x="control point") -> (-x=w639:dbl)
      n408 = Select(t=w639, s=w634, f="control point") -> (s? t:f=w636:dbl)
      n409 = disable-structure shown="Enabled" {
        disable-tunnel: w636 -> [w650 w654]
        disable-tunnel: [w649 w654] -> w635
        frame Enabled {
          n410 = local read "map_track for steering"() -> (w653:dbl[][])
          n411 = Index Array(array=w653, index (col)=1 ("disabled index (col)")) -> (element=w651:dbl[])  [unwired: 1 in]
          n412 = Array Max & Min(array=w651) -> (max value=w645:dbl, min value=w648:dbl)  [unwired: 2 out]
          n413 = Add(x=0.6000000000000001, y=w648) -> (x+y=w647:dbl)
          n414 = In Range and Coerce(upper limit=w645, x=w650, lower limit=w647) -> (coerced(x)=w649:dbl)  [unwired: 1 out]
        }
        frame Disabled {
        }
      }
      n415 = local read "Polynomial Coefficients"() -> (w643:dbl[])
      n416 = call-poly <vilib>:"nth Derivative of Polynomial.vi"("order"=1, "P(x)"=w643) -> ("Nth Derivative of P(x)"=w641:dbl[])  [unwired: 8 in, 1 out]
      n417 = call-poly <vilib>:"Polynomial Evaluation.vi"("P(x)"=w641, "a"=w635) -> ("P(a)"=w638:dbl)  [unwired: 1 out]
    }
    frame #6 {
      n418 = Square(x=w694) -> (x^2=w721:dbl)
      n419 = global read "G_ALL.vi" "CARDATA"() -> (w693:T1)
      n420 = Increment(x=w721) -> (x+1=w719:dbl)
      n421 = local read "Polynomial Coefficients"() -> (w695:dbl[])
      n422 = local read "Polynomial Coefficients"() -> (w680:dbl[])
      n423 = Unbundle By Name(w693) -> ("VS_can"=w692:dbl)
      n424 = Square Root(x=w719) -> (sqrt(x)=w720:dbl)
      n425 = Multiply(x=w720, y=w719) -> (x*y=w718:dbl)
      n426 = Divide(x=w692, y=3.6) -> (x/y=w713:dbl)
      n427 = Absolute Value(x=w713) -> (abs(x)=w716:dbl)
      n428 = call-poly <vilib>:"nth Derivative of Polynomial.vi"("order"=2, "P(x)"=w695) -> ("Nth Derivative of P(x)"=w676:dbl[])  [unwired: 8 in, 1 out]
      n429 = Index Array(array=w680, index=1) -> (element=w678:dbl)
      n430 = call-poly <vilib>:"Polynomial Evaluation.vi"("P(x)"=w676, "a"=w671) -> ("P(a)"=w677:dbl)  [unwired: 1 out]
      n431 = Square(x=w678) -> (x^2=w683:dbl)
      n432 = Inverse Tangent(1:w678) -> (0:w674:dbl)
      n433 = Max & Min(x=w716, y=1.0) -> (max(x,y)=w714:dbl)  [unwired: 1 out]
      n434 = global read "G_ALL.vi" "CARSPEC"() -> (w708:T2)
      n435 = Divide(x=w696, y=w714) -> (x/y=w697:dbl)
      n436 = Divide(x=w718, y=w677) -> (x/y=w700:dbl)
      "R_new" <- w700
      n437 = Negate(x=w674) -> (-x=w673:dbl)
      n438 = Increment(x=w683) -> (x+1=w685:dbl)
      n439 = Unbundle By Name(w708) -> ("ratio_steer"=w710:dbl, "C_Wheel base"=w709:dbl)
      n440 = Select(t=w674, s=w675, f=w673) -> (s? t:f=w698:dbl)
      n441 = Square Root(x=w685) -> (sqrt(x)=w684:dbl)
      n442 = Divide(x=w709, y=w700) -> (x/y=w702:dbl)
      n443 = Multiply(x=w684, y=w685) -> (x*y=w682:dbl)
      n444 = Divide(x=w682, y=w677) -> (x/y=→"R0":dbl)
      n445 = Inverse Tangent(1:w702) -> (0:w704:dbl)
      n446 = Multiply(x=180.0 ("y"), y=w704) -> (x*y=w705:dbl)
      n447 = Divide(x=w705, y=3.141592653589793) -> (x/y=w707:dbl)
      n448 = Multiply(x=w710, y=w707) -> (x*y=w701:dbl)
      n449 = Not A Number/Path/Refnum?(number/path/refnum=w701) -> (NaN/Path/Refnum?=w711:bool)
      n450 = Select(t=0.0, s=w711, f=w701) -> (s? t:f=w699:dbl)
      n451 = Build Array(w699, w698, w697) -> (w690:dbl[])
      "ref" <- w690
      n452 = Multiply(x=w690, y="gain") -> (x*y=w672:dbl[])
      n453 = Add Array Elements(numeric array=w672) -> (sum=w689:dbl)
      "handle 2" <- w689
      n454 = Negate(x=w689) -> (-x=w688:dbl)
      n455 = In Range and Coerce(upper limit=479.0, x=w688, lower limit=-479.0) -> (coerced(x)=w663:dbl, In Range?=w661:bool)
      n456 = Decrement(x="lpf gain 2") -> (x-1=w670:dbl)
      n457 = Multiply(x=w663, y="lpf gain 2") -> (x*y=w668:dbl)
      n458 = case shown="True" w661 {
        frame False {
          n459 = global read "G_ALL.vi" "CARDATA"() -> (w731:T1)
          n460 = global read "G_ALL.vi" "xobs"() -> (w729:cluster{"idx":i32, "x":dbl, "y":dbl, "h":dbl})
          n461 = global read "G_ALL.vi" "Reverse"() -> (w725:bool)
          n462 = Unbundle By Name(w731) -> ("VS_can"=w730:dbl)
          n463 = Unbundle By Name(w729) -> ("idx"=w728:i32)
          n464 = Equal To 0?(x=w730) -> (x = 0?=w726:bool)
          n465 = Not Equal To 0?(x=w728) -> (x != 0?=w727:bool)
          n466 = Not(x=w725) -> (.not. x?=w724:bool)
          n467 = Compound Arithmetic op=AND(w726, w727, w724) -> (w723:bool)
          n468 = case shown="True" w723 {
            selector: w723 -> [_ w732]
            frame False {
            }
            frame True {
              n469 = global write "G_ALL.vi" "Reverse"(w732) -> ()
            }
          }
        }
        frame True {
          n470 = global read "G_ALL.vi" "xobs"() -> (w736:cluster{"idx":i32, "x":dbl, "y":dbl, "h":dbl})
          n471 = global read "G_ALL.vi" "Reverse"() -> (w734:bool)
          n472 = Unbundle By Name(w736) -> ("h"=w737:dbl)
          n473 = Greater?(x=w737, y=5.5) -> (0:w735:bool)
          n474 = And(x=w735, y=w734) -> (x .and. y?=w733:bool)
          n475 = case shown="True" w733 {
            frame False {
            }
            frame True {
              n476 = global write "G_ALL.vi" "Reverse"(FALSE ("Reverse")) -> ()
            }
          }
        }
      }
      n477 = feedback #2(0.0) -> (w669:dbl)
      n478 = Multiply(x=w670, y=w669) -> (x*y=w667:dbl)
      n479 = Subtract(x=w668, y=w667) -> (x-y=w664:dbl)
      "handle" <- w664
      n480 = feedback-in #2(w664) -> ()
      n481 = Merge Signals(w664, w663) -> (→"Waveform Chart 2":dynamicdata)
    }
    frame #7 {
      n482 = local read "dist"() -> (w745:dbl[])
      n483 = local read "Polynomial Coefficients"() -> (w748:dbl[])
      n484 = global write "G_ALL.vi" "Steering dist"(w745) -> ()
      n485 = local read "map_track for speed"() -> (w757:dbl[][])
      n486 = Multiply(x=dbl[] [-3.141592653589793, -3.1315926535897933, -3.121592653589793, -3.1115926535897933, -3.101592653589793, -3.0915926535897933, -3.081592653589793, -3.0715926535897933, -3.061592653589793, -3.0515926535897933, -3.041592653589793, -3.0315926535897932, -3.021592653589793, -3.0115926535897932, -3.001592653589793, -2.991592653589793, -2.981592653589793, -2.971592653589793, -2.961592653589793, -2.951592653589793, -2.941592653589793, -2.931592653589793, -2.921592653589793, -2.911592653589793, -2.901592653589793, -2.891592653589793, -2.8815926535897933, -2.871592653589793, -2.861592653589793, -2.851592653589793, -2.8415926535897933, -2.831592653589793, -2.8215926535897933, -2.811592653589793, -2.8015926535897933, -2.791592653589793, -2.7815926535897932, -2.771592653589793, -2.7615926535897932, -2.751592653589793, -2.741592653589793, -2.731592653589793, -2.721592653589793, -2.711592653589793, -2.701592653589793, -2.691592653589793, -2.681592653589793, -2.671592653589793, -2.661592653589793, -2.651592653589793, -2.641592653589793, -2.6315926535897933, -2.621592653589793, -2.611592653589793, -2.601592653589793, -2.5915926535897933, -2.581592653589793, -2.571592653589793, -2.561592653589793, -2.5515926535897933, -2.541592653589793, -2.5315926535897932, -2.521592653589793, -2.5115926535897932, -2.501592653589793, -2.491592653589793, -2.481592653589793, -2.471592653589793, -2.461592653589793, -2.451592653589793, -2.441592653589793, -2.431592653589793, -2.4215926535897934, -2.411592653589793, -2.401592653589793, -2.391592653589793, -2.3815926535897933, -2.371592653589793, -2.361592653589793, -2.351592653589793, -2.3415926535897933, -2.331592653589793, -2.321592653589793, -2.311592653589793, -2.3015926535897933, -2.291592653589793, -2.2815926535897932, -2.271592653589793, -2.2615926535897932, -2.251592653589793, -2.241592653589793, -2.231592653589793, -2.221592653589793, -2.211592653589793, -2.201592653589793, -2.191592653589793, -2.181592653589793, -2.1715926535897934, -2.161592653589793, -2.151592653589793, -2.141592653589793, -2.1315926535897933, -2.121592653589793, -2.111592653589793, -2.101592653589793, -2.0915926535897933, -2.081592653589793, -2.071592653589793, -2.061592653589793, -2.0515926535897933, -2.041592653589793, -2.031592653589793, -2.021592653589793, -2.0115926535897932, -2.001592653589793, -1.991592653589793, -1.9815926535897932, -1.9715926535897932, -1.9615926535897932, -1.9515926535897932, -1.9415926535897932, -1.9315926535897932, -1.9215926535897931, -1.9115926535897931, -1.9015926535897931, -1.8915926535897931, -1.881592653589793, -1.871592653589793, -1.861592653589793, -1.851592653589793, -1.841592653589793, -1.831592653589793, -1.821592653589793, -1.811592653589793, -1.801592653589793, -1.791592653589793, -1.781592653589793, -1.771592653589793, -1.761592653589793, -1.751592653589793, -1.741592653589793, -1.7315926535897932, -1.7215926535897932, -1.7115926535897932, -1.7015926535897932, -1.6915926535897932, -1.6815926535897932, -1.6715926535897931, -1.6615926535897931, -1.6515926535897931, -1.6415926535897931, -1.631592653589793, -1.621592653589793, -1.611592653589793, -1.601592653589793, -1.591592653589793, -1.581592653589793, -1.571592653589793, -1.561592653589793, -1.551592653589793, -1.541592653589793, -1.531592653589793, -1.521592653589793, -1.511592653589793, -1.501592653589793, -1.491592653589793, -1.481592653589793, -1.4715926535897932, -1.4615926535897932, -1.4515926535897932, -1.4415926535897932, -1.4315926535897932, -1.4215926535897931, -1.4115926535897931, -1.4015926535897931, -1.3915926535897931, -1.381592653589793, -1.371592653589793, -1.361592653589793, -1.351592653589793, -1.341592653589793, -1.331592653589793, -1.321592653589793, -1.311592653589793, -1.301592653589793, -1.291592653589793, -1.281592653589793, -1.271592653589793, -1.261592653589793, -1.251592653589793, -1.241592653589793, -1.231592653589793, -1.2215926535897932, -1.2115926535897932, -1.2015926535897932, -1.1915926535897932, -1.1815926535897932, -1.1715926535897931, -1.1615926535897931, -1.1515926535897931, -1.1415926535897931, -1.1315926535897929, -1.121592653589793, -1.1115926535897929, -1.101592653589793, -1.0915926535897933, -1.081592653589793, -1.0715926535897933, -1.061592653589793, -1.0515926535897933, -1.041592653589793, -1.0315926535897932, -1.021592653589793, -1.0115926535897932, -1.001592653589793, -0.9915926535897932, -0.981592653589793, -0.9715926535897932, -0.961592653589793, -0.9515926535897932, -0.9415926535897929, -0.9315926535897932, -0.9215926535897929, -0.9115926535897931, -0.9015926535897929, -0.8915926535897931, -0.8815926535897929, -0.8715926535897931, -0.8615926535897929, -0.8515926535897931, -0.8415926535897928, -0.8315926535897931, -0.8215926535897933, -0.811592653589793, -0.8015926535897933, -0.791592653589793, -0.7815926535897932, -0.771592653589793, -0.7615926535897932, -0.751592653589793, -0.7415926535897932, -0.731592653589793, -0.7215926535897932, -0.711592653589793, -0.7015926535897932, -0.6915926535897929, -0.6815926535897932, -0.6715926535897929, -0.6615926535897931, -0.6515926535897929, -0.6415926535897931, -0.6315926535897929, -0.6215926535897931, -0.6115926535897929, -0.6015926535897931, -0.5915926535897928, -0.5815926535897931, -0.5715926535897933, -0.561592653589793, -0.5515926535897933, -0.541592653589793, -0.5315926535897932, -0.521592653589793, -0.5115926535897932, -0.501592653589793, -0.4915926535897932, -0.481592653589793, -0.4715926535897932, -0.46159265358979296, -0.45159265358979317, -0.44159265358979294, -0.43159265358979315, -0.4215926535897929, -0.41159265358979313, -0.4015926535897929, -0.3915926535897931, -0.3815926535897929, -0.3715926535897931, -0.36159265358979287, -0.3515926535897931, -0.34159265358979285, -0.33159265358979306, -0.3215926535897933, -0.31159265358979304, -0.30159265358979326, -0.291592653589793, -0.28159265358979324, -0.271592653589793, -0.2615926535897932, -0.251592653589793, -0.2415926535897932, -0.23159265358979297, -0.2215926535897932, -0.21159265358979296, -0.20159265358979317, -0.19159265358979294, -0.18159265358979315, -0.17159265358979292, -0.16159265358979313, -0.1515926535897929, -0.14159265358979312, -0.13159265358979289, -0.1215926535897931, -0.11159265358979287, -0.10159265358979308, -0.09159265358979285, -0.08159265358979306, -0.07159265358979283, -0.061592653589793045, -0.05159265358979326, -0.04159265358979303, -0.03159265358979324, -0.02159265358979301, -0.011592653589793223, -0.0015926535897929917, 0.008407346410206795, 0.018407346410207026, 0.028407346410206813, 0.038407346410207044, 0.04840734641020683, 0.05840734641020706, 0.06840734641020685, 0.07840734641020708, 0.08840734641020687, 0.0984073464102071, 0.10840734641020688, 0.11840734641020711, 0.1284073464102069, 0.13840734641020713, 0.14840734641020692, 0.15840734641020715, 0.16840734641020694, 0.17840734641020717, 0.18840734641020696, 0.19840734641020674, 0.20840734641020697, 0.21840734641020676, 0.228407346410207, 0.23840734641020678, 0.248407346410207, 0.2584073464102068, 0.268407346410207, 0.2784073464102068, 0.28840734641020704, 0.29840734641020683, 0.30840734641020706, 0.31840734641020685, 0.3284073464102071, 0.33840734641020687, 0.3484073464102071, 0.3584073464102069, 0.3684073464102071, 0.3784073464102069, 0.38840734641020713, 0.3984073464102069, 0.40840734641020715, 0.41840734641020694, 0.42840734641020717, 0.43840734641020696, 0.44840734641020674, 0.458407346410207, 0.46840734641020676, 0.478407346410207, 0.4884073464102068, 0.498407346410207, 0.5084073464102068, 0.518407346410207, 0.5284073464102068, 0.538407346410207, 0.5484073464102068, 0.5584073464102071, 0.5684073464102068, 0.5784073464102071, 0.5884073464102069, 0.5984073464102071, 0.6084073464102069, 0.6184073464102071, 0.6284073464102069, 0.6384073464102071, 0.6484073464102069, 0.6584073464102072, 0.6684073464102069, 0.6784073464102072, 0.688407346410207, 0.6984073464102067, 0.708407346410207, 0.7184073464102068, 0.728407346410207, 0.7384073464102068, 0.748407346410207, 0.7584073464102068, 0.768407346410207, 0.7784073464102068, 0.788407346410207, 0.7984073464102068, 0.8084073464102071, 0.8184073464102068, 0.8284073464102071, 0.8384073464102069, 0.8484073464102071, 0.8584073464102069, 0.8684073464102067, 0.8784073464102073, 0.8884073464102071, 0.8984073464102069, 0.9084073464102067, 0.9184073464102074, 0.9284073464102072, 0.938407346410207, 0.9484073464102067, 0.9584073464102065, 0.9684073464102072, 0.978407346410207, 0.9884073464102068, 0.9984073464102066, 1.0084073464102072, 1.018407346410207, 1.0284073464102068, 1.0384073464102066, 1.0484073464102073, 1.058407346410207, 1.0684073464102068, 1.0784073464102066, 1.0884073464102073, 1.098407346410207, 1.1084073464102069, 1.1184073464102067, 1.1284073464102073, 1.1384073464102071, 1.148407346410207, 1.1584073464102067, 1.1684073464102074, 1.1784073464102072, 1.188407346410207, 1.1984073464102067, 1.2084073464102074, 1.2184073464102072, 1.228407346410207, 1.2384073464102068, 1.2484073464102066, 1.2584073464102072, 1.268407346410207, 1.2784073464102068, 1.2884073464102066, 1.2984073464102073, 1.308407346410207, 1.3184073464102068, 1.3284073464102066, 1.3384073464102073, 1.348407346410207, 1.3584073464102069, 1.3684073464102067, 1.3784073464102073, 1.3884073464102071, 1.398407346410207, 1.4084073464102067, 1.4184073464102074, 1.4284073464102072, 1.438407346410207, 1.4484073464102067, 1.4584073464102074, 1.4684073464102072, 1.478407346410207, 1.4884073464102068, 1.4984073464102066, 1.5084073464102072, 1.518407346410207, 1.5284073464102068, 1.5384073464102066, 1.5484073464102073, 1.558407346410207, 1.5684073464102068, 1.5784073464102066, 1.5884073464102073, 1.598407346410207, 1.6084073464102069, 1.6184073464102067, 1.6284073464102073, 1.6384073464102071, 1.648407346410207, 1.6584073464102067, 1.6684073464102074, 1.6784073464102072, 1.688407346410207, 1.6984073464102067, 1.7084073464102074, 1.7184073464102072, 1.728407346410207, 1.7384073464102068, 1.7484073464102066, 1.7584073464102072, 1.768407346410207, 1.7784073464102068, 1.7884073464102066, 1.7984073464102073, 1.808407346410207, 1.8184073464102068, 1.8284073464102066, 1.8384073464102073, 1.848407346410207, 1.8584073464102069, 1.8684073464102067, 1.8784073464102073, 1.8884073464102071, 1.898407346410207, 1.9084073464102067, 1.9184073464102074, 1.9284073464102072, 1.938407346410207, 1.9484073464102067, 1.9584073464102074, 1.9684073464102072, 1.978407346410207, 1.9884073464102068, 1.9984073464102066, 2.0084073464102072, 2.018407346410207, 2.028407346410207, 2.0384073464102066, 2.0484073464102073, 2.058407346410207, 2.068407346410207, 2.0784073464102066, 2.0884073464102073, 2.098407346410207, 2.108407346410207, 2.1184073464102067, 2.1284073464102073, 2.138407346410207, 2.148407346410207, 2.1584073464102067, 2.1684073464102074, 2.178407346410207, 2.188407346410207, 2.1984073464102067, 2.2084073464102074, 2.218407346410207, 2.228407346410207, 2.2384073464102068, 2.2484073464102066, 2.2584073464102072, 2.268407346410207, 2.278407346410207, 2.2884073464102066, 2.2984073464102073, 2.308407346410207, 2.318407346410207, 2.3284073464102066, 2.3384073464102073, 2.348407346410207, 2.358407346410207, 2.3684073464102067, 2.3784073464102073, 2.388407346410207, 2.398407346410207, 2.4084073464102067, 2.4184073464102074, 2.428407346410207, 2.438407346410207, 2.4484073464102067, 2.4584073464102074, 2.468407346410207, 2.478407346410207, 2.4884073464102068, 2.4984073464102066, 2.5084073464102072, 2.518407346410207, 2.528407346410207, 2.5384073464102066, 2.5484073464102073, 2.558407346410207, 2.568407346410207, 2.5784073464102066, 2.5884073464102073, 2.598407346410207, 2.608407346410207, 2.6184073464102067, 2.6284073464102073, 2.638407346410207, 2.648407346410207, 2.6584073464102067, 2.6684073464102074, 2.678407346410207, 2.688407346410207, 2.6984073464102067, 2.7084073464102074, 2.718407346410207, 2.728407346410207, 2.7384073464102068, 2.7484073464102066, 2.7584073464102072, 2.768407346410207, 2.778407346410207, 2.7884073464102066, 2.7984073464102073, 2.808407346410207, 2.818407346410207, 2.8284073464102066, 2.8384073464102073, 2.848407346410207, 2.858407346410207, 2.8684073464102067, 2.8784073464102073, 2.888407346410207, 2.898407346410207, 2.9084073464102067, 2.9184073464102074, 2.928407346410207, 2.938407346410207, 2.9484073464102067, 2.9584073464102074, 2.968407346410207, 2.978407346410207, 2.9884073464102068, 2.9984073464102075, 3.0084073464102072, 3.018407346410207, 3.028407346410207, 3.0384073464102066, 3.0484073464102073, 3.058407346410207, 3.068407346410207, 3.0784073464102066, 3.0884073464102073, 3.098407346410207, 3.108407346410207, 3.1184073464102067, 3.1284073464102073, 3.138407346410207] ("theta"), y=2.0) -> (x*y=w741:dbl[])
      n487 = local read "R0"() -> (w749:dbl)
      n488 = call-poly <vilib>:"Polynomial Evaluation.vi"("P(x)"=w748, "A"=w741) -> ("P(A)"=w744:dbl[])  [unwired: 1 out]
      n489 = call "Convert to Dynamic Data3"("Array"=w741) -> ("Dynamic Data Type"=w752:dynamicdata)  [unwired: 3 in]
      n490 = Index Array(array=w757, index (col) #1=0 ("disabled index (col)")) -> (element #1=w755:dbl[], element #2=w743:dbl[])  [unwired: 3 in]
      n491 = Build Array (concatenate)(w749, w748) -> (w750:dbl[])
      n492 = call "Convert to Dynamic Data"("Array"=w755) -> ("Dynamic Data Type"=w754:dynamicdata)  [unwired: 3 in]
      n493 = call "Convert to Dynamic Data2"("Array"=w743) -> ("Dynamic Data Type"=w753:dynamicdata)  [unwired: 3 in]
      n494 = call "Convert to Dynamic Data4"("Array"=w744) -> ("Dynamic Data Type"=w751:dynamicdata)  [unwired: 3 in]
      n495 = global write "G_ALL.vi" "Steering coeff"(w750) -> ()
      n496 = Merge Signals(w754, w751) -> (w746:dynamicdata)
      n497 = Merge Signals(w753, w752) -> (w747:dynamicdata)
      n498 = call "Build XY Graph"("Y Input"=w747, "X Input"=w746) -> ("XY Graph"=→"XY Graph":cluster{"X":dbl[], "Y":dbl[]}[])  [unwired: 8 in, 1 out]
    }
  }
